vi "AddLimit.vi"(7 "ComparisonType":T1, 8 "error in":errorcluster, 9 "HigherBond":i64, 10 "LowerBound":i64, 11 "IntergerMeasure in":refnum<class "IntegerMeasure.lvclass">) -> (0 "error out":errorcluster, 2 "IntegerMeasureLimit":refnum<class "IntegerMeasureLimit.lvclass">, 3 "IntergerMeasure out":refnum<class "IntegerMeasure.lvclass">)   [LabVIEW 2021, in "ProligentXMLGenerator.lvlib" / "IntegerMeasure.lvclass"]
doc: "Add a MeasureLimit element.\n\nThe limit expression associated with the measure."
uses:
  IntegerMeasure.lvclass
  IntegerMeasure.lvclass/IntegerMeasure.ctl
  MeasureLimit/MeasureLimit.lvclass
  IntegerMeasureLimit/IntegerMeasureLimit.lvclass
  RangeMeasureLimit/ComparisonType.ctl
  RangeMeasureLimit/RangeMeasureLimit.lvclass
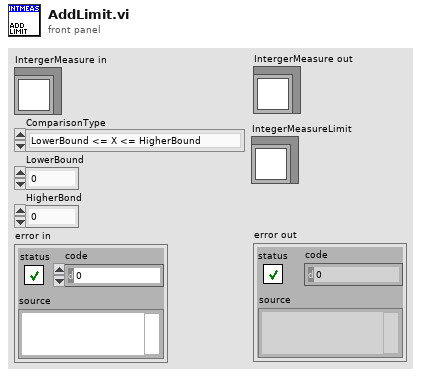
[diagram p1: front panel]
types:
  T1 = typedef "ProligentXMLGenerator.lvlib/RangeMeasureLimit.lvclass/ComparisonType.ctl" = enum16{"LowerBound <= X <= HigherBound", "LowerBound < X <= HigherBound", "LowerBound <= X < HigherBound", "LowerBound < X < HigherBound", "LowerBound <= X", "LowerBound < X", "X <= HigherBound", "X < HigherBound", "X == HigherBound", "X != HigherBound", "X <= LowerBound OR HigherBound <= X", "X < LowerBound OR HigherBound <= X", "X <= LowerBound OR HigherBound < X", "X < LowerBound OR HigherBound < X"}
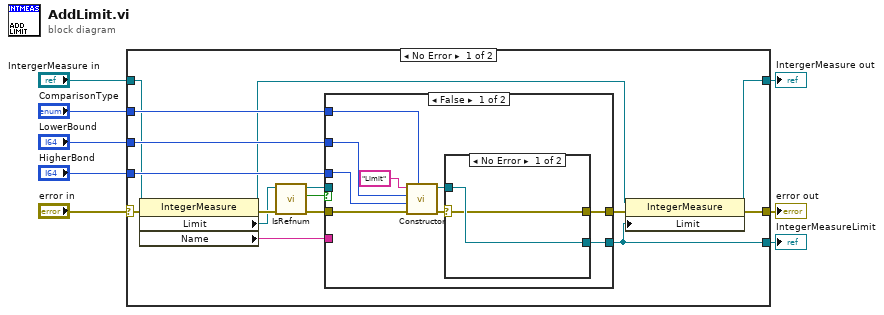
[diagram p0: block diagram]
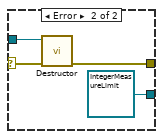
[diagram p2: hidden frame]
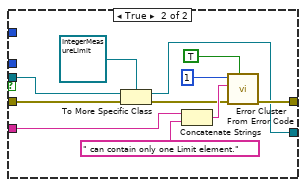
[diagram p3: hidden frame]
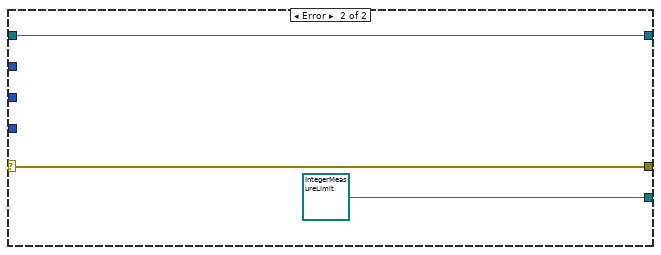
[diagram p4: hidden frame]
diagram:
  n1 = case shown="No Error" "error in" {
    selector: "error in" -> [w23 w52]
    tunnel: [w13 refnum<class "IntegerMeasureLimit.lvclass"> refnum ("ProligentResultProcessor:IntegerMeasureLimit")] -> w4
    tunnel: [w15 w52] -> w7
    tunnel: "IntergerMeasure in" -> [w12 w53]
    tunnel: [w14 w53] -> w5
    tunnel: "ComparisonType" -> [w18 _]
    tunnel: "LowerBound" -> [w17 _]
    tunnel: "HigherBond" -> [w16 _]
    frame No Error {
      n2 = property class="IntegerMeasure"(reference=w12, error in=w23) -> (reference out=w11:refnum<class "IntegerMeasure.lvclass">, error out=w22:errorcluster, "Limit"=w10:refnum<class "MeasureLimit.lvclass">, "Name"=w21:string)
      n3 = call "IsRefnum.vi"("error in"=w22, "MeasureLimit in"=w10) -> ("error out"=w20:errorcluster, "IsRefnum"=w19:bool, "MeasureLimit out"=w9:refnum<class "MeasureLimit.lvclass">)  [unwired: 7 in]
      n4 = case shown="False" w19 {
        tunnel: w20 -> [w27 w43]
        tunnel: [w33 w46] -> w24
        tunnel: [w32 w41] -> w13
        tunnel: w21 -> [_ w45]
        tunnel: w18 -> [w31 _]
        tunnel: w17 -> [w30 _]
        tunnel: w16 -> [w28 _]
        tunnel: w9 -> [_ w44]
        frame False {
          n5 = call "Constructor.vi"("ComparisonType"=w31, "error in"=w27, "HigherBond"=w28, "LowerBound"=w30, "Name"="Limit") -> ("error out"=w26:errorcluster, "IntegerMeasureLimit"=w25:refnum<class "IntegerMeasureLimit.lvclass">)  [unwired: 5 in]
          n6 = case shown="No Error" w26 {
            selector: w26 -> [w34 w39]
            tunnel: w25 -> [w35 w37]
            tunnel: [w34 w38] -> w33
            tunnel: [w35 refnum<class "IntegerMeasureLimit.lvclass"> refnum ("ProligentResultProcessor:IntegerMeasureLimit")] -> w32
            frame No Error {
            }
            frame Error {
              n7 = call "Destructor.vi"("error in"=w39, "IntegerMeasureLimit"=w37) -> ("error out"=w38:errorcluster)  [unwired: 9 in]
            }
          }
        }
        frame True {
          n8 = To More Specific Class(target class=refnum<class "IntegerMeasureLimit.lvclass"> refnum ("ProligentResultProcessor:IntegerMeasureLimit"), reference=w44, error in=w43) -> (specific class reference=w41:refnum<class "IntegerMeasureLimit.lvclass">, error out=w42:errorcluster)
          n9 = Concatenate Strings(w45, " can contain only one Limit element." ("string")) -> (w50:string)
          n10 = call <vilib>:"Error Cluster From Error Code.vi"("show call chain? (False)"=TRUE, "error in (no error)"=w42, "error message (\"\")"=w50, "error code (0)"=1) -> ("error out"=w46:errorcluster)  [unwired: 5 in]
        }
      }
      n11 = property class="IntegerMeasure"(reference=w11, error in=w24, "Limit"=w13) -> (reference out=w14:refnum<class "IntegerMeasure.lvclass">, error out=w15:errorcluster)
    }
    frame Error {
    }
  }
  "error out" <- w7
  "IntergerMeasure out" <- w5
  "IntegerMeasureLimit" <- w4
